vi "daq.io Machine Example.vi"(8 "error in":errorcluster) -> (0 "error out":errorcluster)   [LabVIEW 2013, in "daqio minimal.lvlib"]
doc: "This interactive example demonstrates how a device or machine could continuously publish data to daq.io. When correct user credentials are given, it will log on to daq.io, autocreate all device settings if required and will update time series values continuously. When changing the tag values (or Tags), these will be updated as well. When firing an Event, it will become visible on the daq.io events page. \n\nRefer to the Embedded example for an example that can easily be run on a RIO platform continuously."
uses:
  daqio minimal.lvlib
  _typedefs/update-button.ctl
  _typedefs/trigger-button.ctl
  _typedefs/exmpl_overlay_mask.ctl
  _typedefs/dashboard-button.ctl
  _typedefs/waveform-button.ctl
  _typedefs/exmpl-states.ctl
  _typedefs/daqio-Credentials.ctl
  _typedefs/daqio-Type.ctl
  <vilib>/httpClient/ClientHandle.ctl
  <vilib>/Platform/browser.llb/Open URL in Default Browser (string).vi
  _subs/daqio_Write_Multiple_single_Timestamp.vi
  _subs/daqio_Write_Waveform.vi
  <vilib>/httpClient/LabVIEWHTTPClient.lvlib
  <vilib>/measure/NI_MABase.lvlib
panel:
  out "overlay mask":T1
  in  "Create Waveform":T2
  in  "Create Dashboard":T3
  out "Log":string[](array[string])
  in  "Stop":bool
  in  "Fire Event":T4
  in  "Select Event":u16(ring) items=["Safety Hood Status", "Manual Operation", "Shutting Down"]
  out "Time Stamp sent":timestamp
  in  "Event Data":string
  in  "Update Tags":T5
  out "connected to daq.io":bool
  in  "Sign up link":bool caption="Boolean"
  out "Speed (RPM)":dbl(knob) scale=0.0..2000.0
  out "Temperature Data":dbl(graph)
  out "RAM":dbl(slide) scale=0.0..100.0
  out "CPU":dbl(slide) scale=0.0..100.0
  in  "Setpoint\n(set manually)":dbl(knob) scale=0.0..100.0
  in  "Value 3":string="1234-abc"
  in  "Value 2":string="XYZ 3000 Plus"
  in  "Tag 3":string="Serial Number"
  in  "Tag 2":string="Type"
  in  "Value 1":string="47.615459, -122.323804"
  in  "Tag 1":string="Location"
  out "Device Key":string
  in  "Log On":bool
  in  "User Name (your email)":string
  in  "Password":string
  out "Dashboard URL - copy and open in your web browser":string
  # "Get your free account at daq.io first: sign up at"
  # "This Machine"
  # "(autogenerated in this example)"
  # "Device Tags"
  # "Use device tags to describe \nspecific parameters for each\ndevice. These can include the \nlocation, the serial number or\nother machine or location-\nspecific information. These\nfields are fully user-defined."
  # "Device Events"
  # "Use device events to signal\nany local event to daq.io. These\ncould include mechanical events\n(e.g. \"safety latch released\") or \nany change on the device that\nneeds to be tracked."
  # "Device Live Data Channels"
  # "Use device channels to transfer\ntime series data. All channels \nof the device will be visible in \nthe online data viewer. You \ncan build your own dashboard \nin the webbrowser and link it\nto exisiting channels. Clicking\n\"Create Dashboard\" will\ngenerate a dashboard \nfor this example."
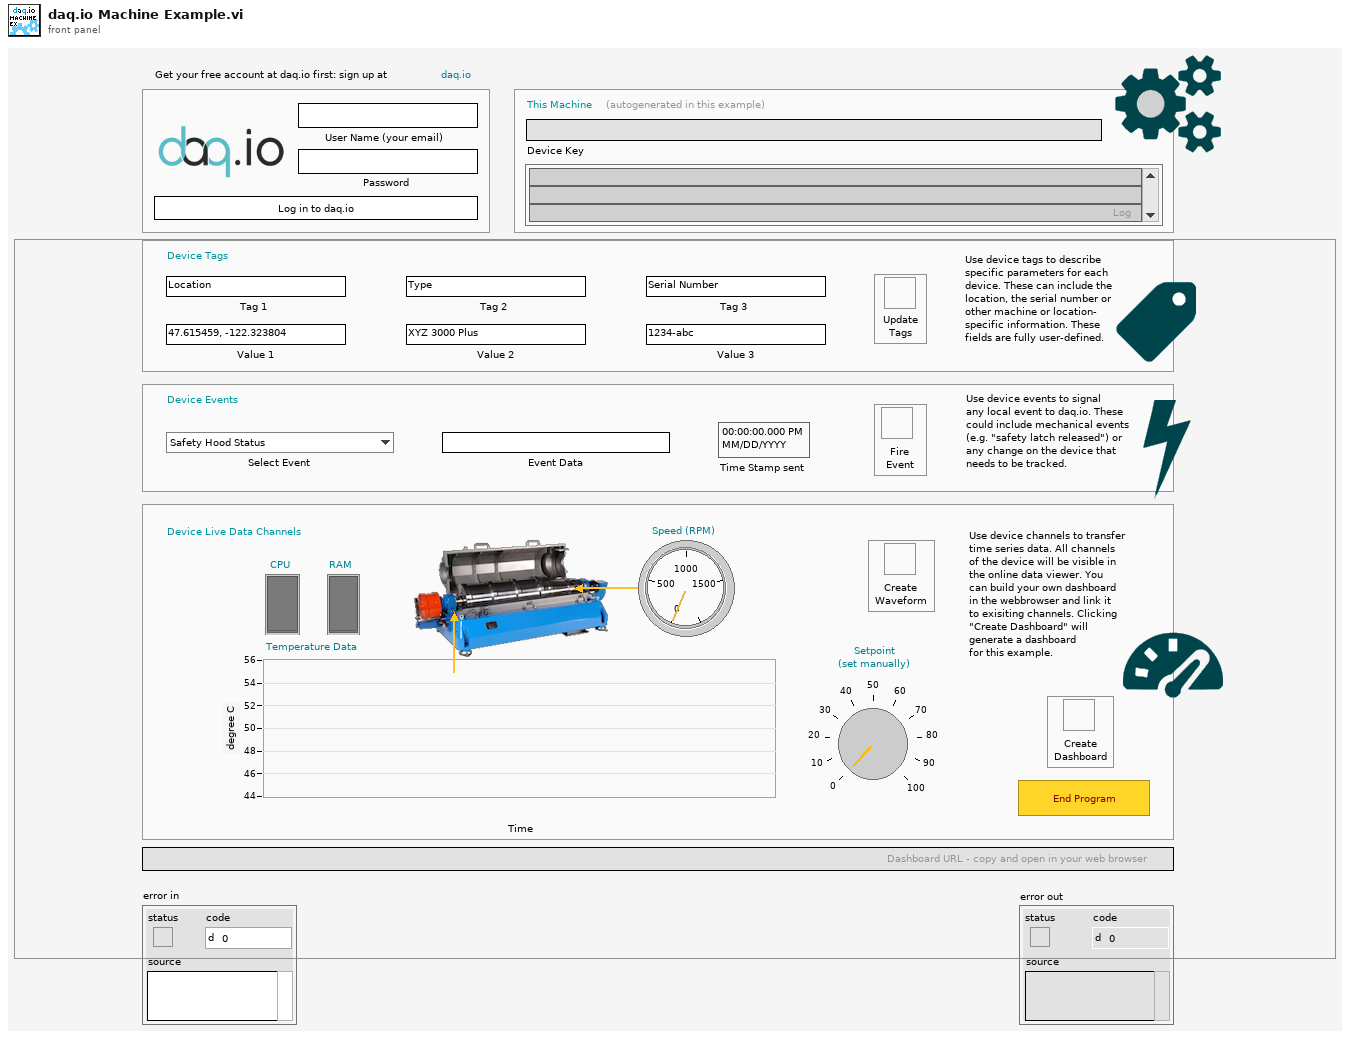
[diagram p1: front panel]
types:
  T1 = typedef "daqio minimal.lvlib/exmpl_overlay_mask.ctl" = bool
  T2 = typedef "daqio minimal.lvlib/waveform-button.ctl" = bool
  T3 = typedef "daqio minimal.lvlib/dashboard-button.ctl" = bool
  T4 = typedef "daqio minimal.lvlib/trigger-button.ctl" = bool
  T5 = typedef "daqio minimal.lvlib/update-button.ctl" = bool
  T6 = typedef "daqio minimal.lvlib/exmpl-states.ctl" = enum16{"idle", "time series", "fire events", "update tags", "end program", "create waveform", "create dashboard"}
  T7 = typedef "daqio minimal.lvlib/daqio-Credentials.ctl" = cluster{"User Name (email)":string, "Password":string}
  T8 = typedef "daqio minimal.lvlib/daqio-Type.ctl" = cluster{"daq.io ref":T9, "daq.io API Base":string, "Device Key":string, "Account ID":string, "online":bool, "SSL":bool, "buffer":bool}
  T9 = typedef "LabVIEWHTTPClient.lvlib/ClientHandle.ctl" = refnum<k1>
  T10 = enum8{"Enabled", "Disabled", "Disabled and Grayed Out"}
  T11 = enum16{"Sine Wave", "Triangle Wave", "Square Wave", "Sawtooth Wave"}
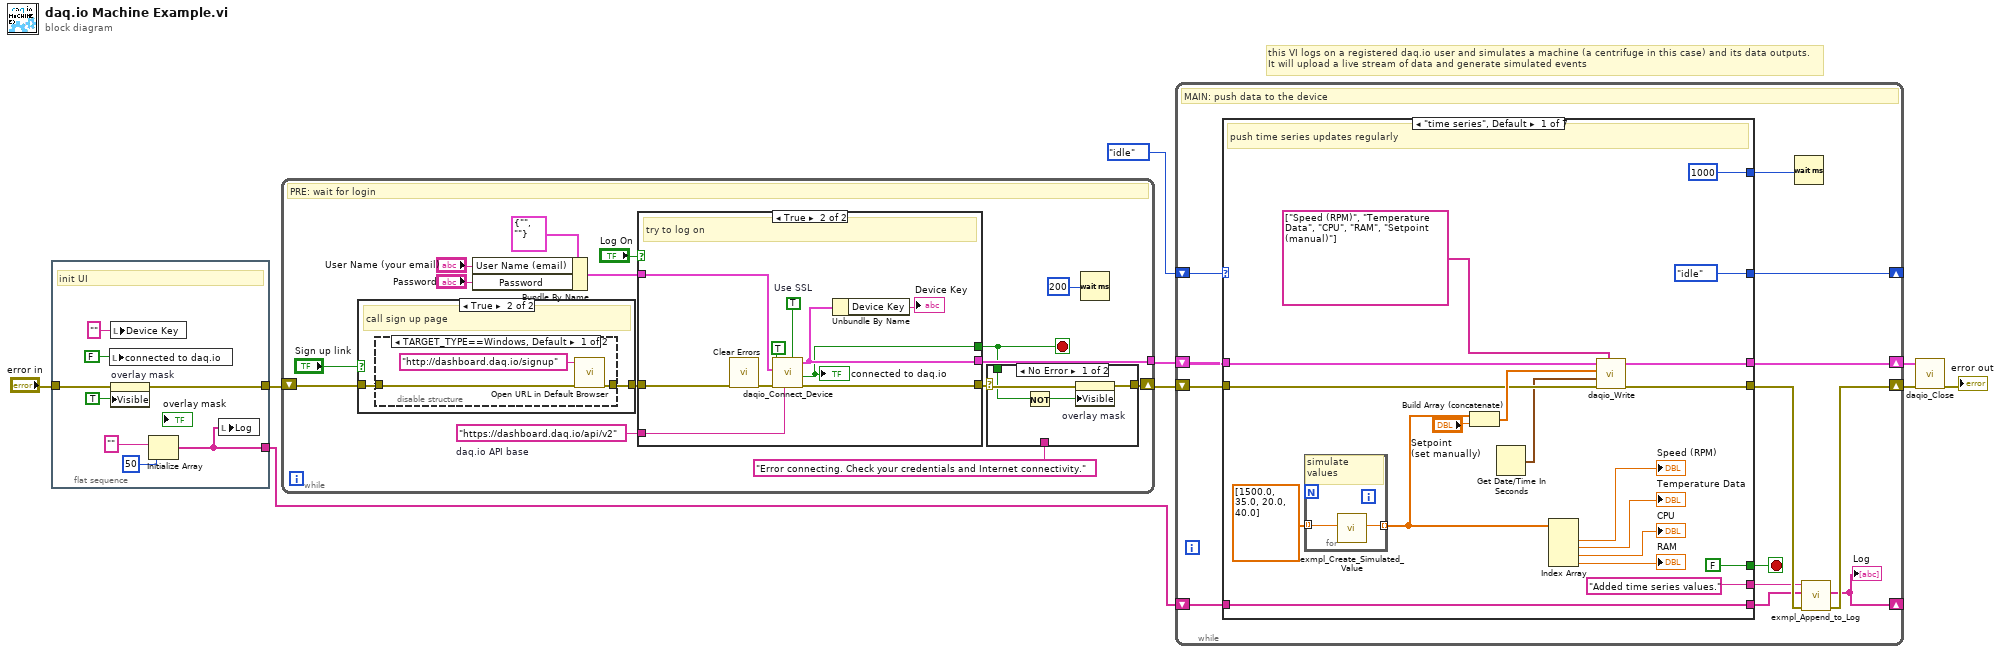
[diagram p0: block diagram]
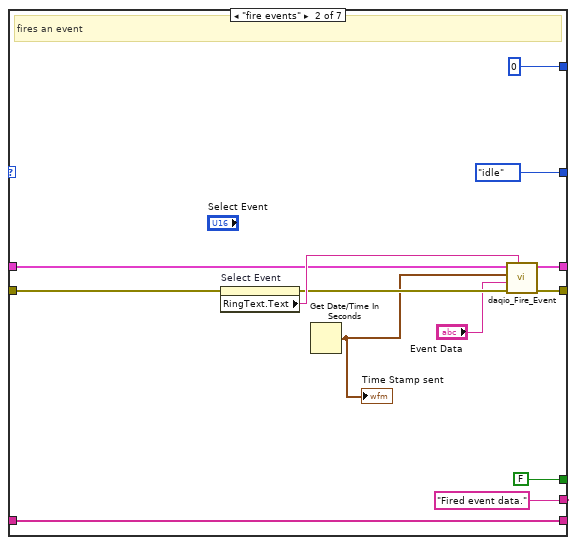
[diagram p2: hidden frame]
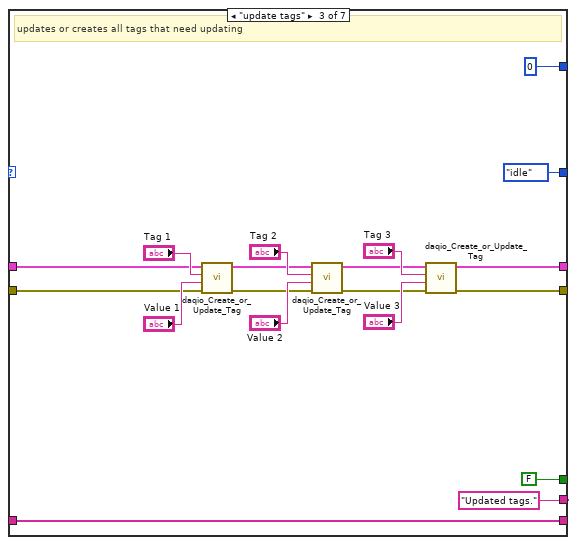
[diagram p3: hidden frame]
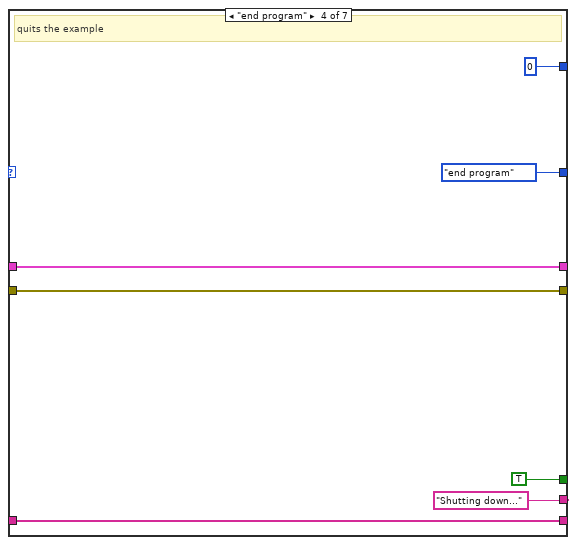
[diagram p4: hidden frame]
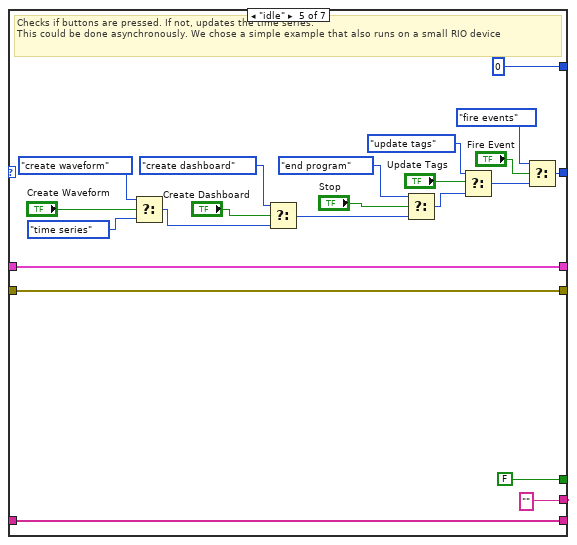
[diagram p5: hidden frame]
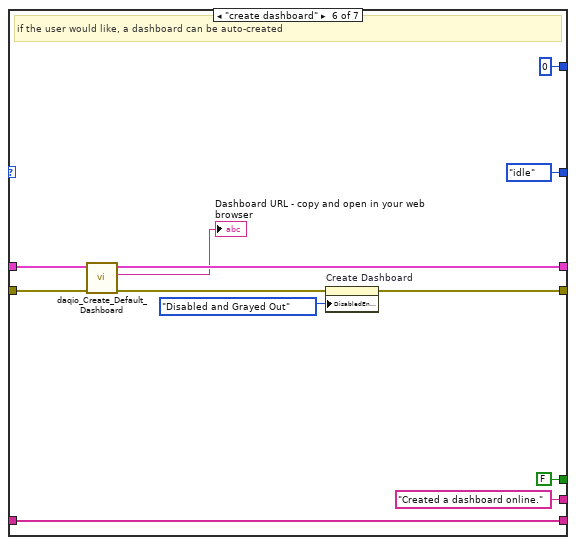
[diagram p6: hidden frame]
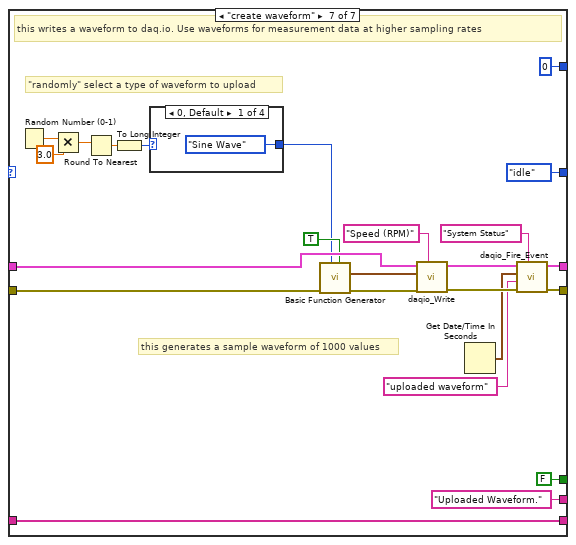
[diagram p7: hidden frame]
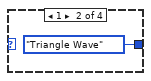
[diagram p8: hidden frame]
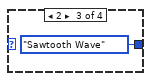
[diagram p9: hidden frame]
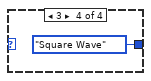
[diagram p10: hidden frame]
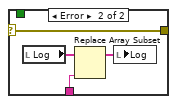
[diagram p11: hidden frame]
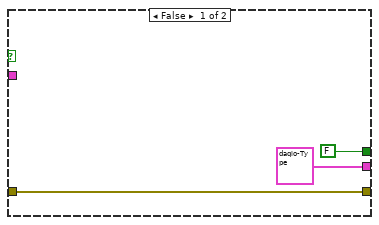
[diagram p14: hidden frame]
diagram:
  # "this VI logs on a registered daq.io user and simulates a machine (a centrifuge in this case) and its data outputs. \nIt will upload a live stream of data and generate simulated events"
  n1 = flat-sequence {
    tunnel: [w14] -> w6
    tunnel: "error in" -> [w15]
    tunnel: [w10] -> w1
    frame #0 {
      # "init UI"
      n2 = local write "connected to daq.io"(FALSE ("connected to daq.io")) -> ()
      n3 = local write "Device Key"("" ("log")) -> ()
      n4 = property on="overlay mask" class="Bool (strict)"(error in=w15, "Visible"=TRUE) -> (error out=w14:errorcluster)  [unwired: 1 in, 1 out]
      n5 = Initialize Array("" ("log"), 50 ("dimension size")) -> (w10:string[])
      n6 = local write "Log"(w10) -> ()
    }
  }
  n7 = while {
    shift-right: [w20] -> w4
    shift-left: w6 -> [w25]
    tunnel: [w27] -> w5
    stop <- w19 stop-if-true
    w18 = "https://dashboard.daq.io/api/v2"  # daq.io API base
    # "PRE: wait for login"
    n8 = case shown="True" "Sign up link" {
      tunnel: w25 -> [w41 w43]
      tunnel: [w41 w42] -> w24
      frame False {
      }
      frame True {
        # "call sign up page"
        n9 = disable-structure shown="TARGET_TYPE==Windows, Default" {
          disable-tunnel: w43 -> [w45 w47]
          disable-tunnel: [w44 w47] -> w42
          frame condition #0 (active) {
            n10 = call-poly <vilib>:"Open URL in Default Browser.vi"("error in (no error)"=w45, "URL"="http://dashboard.daq.io/signup") -> ("error out"=w44:errorcluster)  [unwired: 4 in, 1 out]
          }
          frame condition #1 {
          }
        }
      }
    }
    n11 = Bundle By Name(cluster=T7 {"User Name (email)"="", "Password"=""} ("daq.io Credentials"), "User Name (email)"="User Name (your email)", "Password"="Password") -> (w26:T7)
    n12 = case shown="True" "Log On" {
      tunnel: [T8 {"daq.io ref"=refnum, "daq.io API Base"="http://dashboard.daq.io/api/v1", "Device Key"="", "Account ID"="", "online"=FALSE, "SSL"=FALSE, "buffer"=FALSE} ("daq.io type out") w57] -> w27
      tunnel: [w48 w60] -> w21
      tunnel: w24 -> [w48 w59]
      tunnel: w18 -> [_ w58]
      tunnel: w26 -> [_ w51]
      tunnel: [FALSE ("connected successfully?") w55] -> w19
      frame False {
      }
      frame True {
        w52 = TRUE  # Use SSL
        # "try to log on"
        n13 = call <vilib>:"Clear Errors.vi"("error in (no error)"=w59) -> ("error out"=w54:errorcluster)  [unwired: 6 in]
        n14 = call "daqio_Connect_Device.vi"("Use SSL"=w52, "daq.io API base"=w58, "error in (no error)"=w54, "Credentials"=w51, "Use System Status Event?"=TRUE) -> ("error out"=w60:errorcluster, "connected successfully?"=w55:bool, "daq.io type out"=w57:T8)  [unwired: 4 in]
        "connected to daq.io" <- w55
        n15 = Unbundle By Name(w57) -> ("Device Key"=→"Device Key":string)
      }
    }
    n16 = case shown="No Error" w21 {
      selector: w21 -> [w35 w37]
      tunnel: "Error connecting. Check your credentials and Internet connectivity." ("new element/subarray") -> [_ w38]
      tunnel: [w36 w37] -> w20
      tunnel: w19 -> [w34 _]
      frame No Error {
        n17 = Not(x=w34) -> (.not. x?=w33:bool)
        n18 = property on="overlay mask" class="Bool (strict)"(error in=w35, "Visible"=w33) -> (error out=w36:errorcluster)  [unwired: 1 in, 1 out]
      }
      frame Error {
        n19 = local read "Log"() -> (w40:string[])
        n20 = Replace Array Subset(array=w40, new element=w38) -> (w39:string[])  [unwired: 1 in]
        n21 = local write "Log"(w39) -> ()
      }
    }
    n22 = Wait (ms)(milliseconds to wait=u32 200) -> ()  [unwired: 1 out]
  }
  n23 = while {
    shift-right: [w64] -> w9
    shift-left: w4 -> [w72]
    shift-right: [w71] -> w3
    shift-left: w5 -> [w73]
    shift-right: [w69] -> _
    shift-left: exmpl-states."idle" -> [w70]
    shift-right: [w61] -> _
    shift-left: w1 -> [w66]
    stop <- w68 stop-if-true
    # "MAIN: push data to the device"
    n24 = case shown="\"time series\", Default" w70 {
      tunnel: w73 -> [w80 w104 w116 w131 w136 w162 w190]
      tunnel: w72 -> [w77 w103 w115 w130 w135 w161 w187]
      tunnel: [w74 w101 w113 w131 w136 w160 w180] -> w71
      tunnel: [w75 w102 w114 w130 w135 w157 w179] -> w65
      tunnel: [exmpl-states."idle" exmpl-states."idle" exmpl-states."idle" exmpl-states."end program" w152 exmpl-states."idle" exmpl-states."idle"] -> w69
      tunnel: [FALSE FALSE FALSE TRUE FALSE FALSE FALSE] -> w68
      tunnel: [u32 1000 ("milliseconds to wait") u32 0 ("milliseconds to wait") u32 0 ("milliseconds to wait") u32 0 ("milliseconds to wait") u32 0 ("milliseconds to wait") u32 0 ("milliseconds to wait") u32 0 ("milliseconds to wait")] -> w67
      tunnel: ["Added time series values." ("log") "Fired event data." ("log") "Updated tags." ("log") "Shutting down..." ("log") "" ("log") "Created a dashboard online." ("log") "Uploaded Waveform." ("log")] -> w63
      tunnel: w66 -> [w82 w96 w108 w127 w144 w167 w191]
      tunnel: [w82 w96 w108 w127 w144 w167 w191] -> w62
      frame "time series", Default {
        # "push time series updates regularly"
        n25 = for {
          tunnel: [w94] -> w91 mode=indexing
          tunnel: dbl[] [1500.0, 35.0, 20.0, 40.0] -> [w93] mode=indexing
          # "simulate\nvalues"
          n26 = call "exmpl_Create_Simulated_Value.vi"("offset"=w93) -> ("Numeric"=w94:dbl)  [unwired: 9 in, 1 out]
        }
        n27 = Build Array (concatenate)(w91, "Setpoint\n(set manually)") -> (w78:dbl[])
        n28 = Get Date/Time In Seconds() -> (seconds since 1Jan1904=w76:timestamp)
        n29 = Index Array(array=w91) -> (element #1=→"Speed (RPM)":dbl, element #2=→"Temperature Data":dbl, element #3=→"CPU":dbl, element #4=→"RAM":dbl)  [unwired: 4 in]
        n30 = call-poly "daqio_Write.vi"("daq.io Device Channel Keys"=string[] ["Speed (RPM)", "Temperature Data", "CPU", "RAM", "Setpoint (manual)"], "error in (no error)"=w77, "Timestamp"=w76, "Values"=w78, "daq.io type in"=w80) -> ("error out"=w75:errorcluster, "daq.io type out"=w74:T8)  [unwired: 5 in]
      }
      frame "fire events" {
        # "fires an event"
        n31 = property on="Select Event" class="Ring (strict)"(error in=w103) -> (error out=w106:errorcluster, "RingText.Text"=w107:string)  [unwired: 1 in, 1 out]
        n32 = Get Date/Time In Seconds() -> (seconds since 1Jan1904=w95:timestamp)
        "Time Stamp sent" <- w95
        n33 = call "daqio_Fire_Event.vi"("Event Key"=w107, "error in (no error)"=w106, "Event Value"="Event Data", "Event Date and Time"=w95, "daq.io type in"=w104) -> ("error out"=w102:errorcluster, "daq.io type out"=w101:T8)  [unwired: 5 in]
      }
      frame "update tags" {
        # "updates or creates all tags that need updating"
        n34 = call "daqio_Create_or_Update_Tag.vi"("error in (no error)"=w115, "Tag Value"="Value 1", "Tag Key"="Tag 1", "daq.io type in"=w116) -> ("error out"=w120:errorcluster, "daq.io type out"=w117:T8)  [unwired: 5 in, 1 out]
        n35 = call "daqio_Create_or_Update_Tag.vi"("error in (no error)"=w120, "Tag Value"="Value 2", "Tag Key"="Tag 2", "daq.io type in"=w117) -> ("error out"=w119:errorcluster, "daq.io type out"=w118:T8)  [unwired: 5 in, 1 out]
        n36 = call "daqio_Create_or_Update_Tag.vi"("error in (no error)"=w119, "Tag Value"="Value 3", "Tag Key"="Tag 3", "daq.io type in"=w118) -> ("error out"=w114:errorcluster, "daq.io type out"=w113:T8)  [unwired: 5 in, 1 out]
      }
      frame "end program" {
        # "quits the example"
      }
      frame "idle" {
        # "Checks if buttons are pressed. If not, updates the time series. \nThis could be done asynchronously. We chose a simple example that also runs on a small RIO device"
        n37 = Select(t=exmpl-states."create waveform", s="Create Waveform", f=exmpl-states."time series") -> (s? t:f=w138:T6)
        n38 = Select(t=exmpl-states."create dashboard", s="Create Dashboard", f=w138) -> (s? t:f=w141:T6)
        n39 = Select(t=exmpl-states."end program", s="Stop", f=w141) -> (s? t:f=w146:T6)
        n40 = Select(t=exmpl-states."update tags", s="Update Tags", f=w146) -> (s? t:f=w153:T6)
        n41 = Select(t=exmpl-states."fire events", s="Fire Event", f=w153) -> (s? t:f=w152:T6)
      }
      frame "create dashboard" {
        # "if the user would like, a dashboard can be auto-created"
        n42 = call "daqio_Create_Default_Dashboard.vi"("error in"=w161, "daq.io type in"=w162) -> ("error out"=w158:errorcluster, "Dashboard URL"=→"Dashboard URL - copy and open in your web browser":string, "daq.io type out"=w160:T8)  [unwired: 7 in]
        n43 = property on="Create Dashboard" class="Bool"(error in=w158, "DisabledEnum"=T10."Disabled and Grayed Out" ("Disabled")) -> (error out=w157:errorcluster)  [unwired: 1 in, 1 out]
      }
      frame "create waveform" {
        # "\"randomly\" select a type of waveform to upload"
        # "this generates a sample waveform of 1000 values"
        # "this writes a waveform to daq.io. Use waveforms for measurement data at higher sampling rates"
        n44 = Random Number (0-1)() -> (number: 0 to 1=w173:dbl)
        n45 = Multiply(x=w173, y=3.0) -> (x*y=w171:dbl)
        n46 = Round To Nearest(number=w171) -> (nearest integer value=w170:dbl)
        n47 = To Long Integer(number=w170) -> (32bit integer=w169:i32)
        n48 = case shown="0, Default" w169 {
          tunnel: [T11."Sine Wave" ("signal type") T11."Triangle Wave" ("signal type") T11."Sawtooth Wave" ("signal type") T11."Square Wave" ("signal type")] -> w168
          frame 0, Default {
          }
          frame 1 {
          }
          frame 2 {
          }
          frame 3 {
          }
        }
        n49 = call <vilib>:"Basic Function Generator.vi"("reset signal"=TRUE, "signal type"=w168, "error in (no error)"=w187) -> ("error out"=w189:errorcluster, "signal out"=w188:waveform(dbl))  [unwired: 6 in, 1 out]
        n50 = call-poly "daqio_Write.vi"("daq.io Device Channel Key"="Speed (RPM)" ("daq.io Device Channel"), "error in (no error)"=w189, "Waveform"=w188, "daq.io type in"=w190) -> ("error out"=w178:errorcluster, "daq.io type out"=w181:T8)  [unwired: 6 in]
        n51 = Get Date/Time In Seconds() -> (seconds since 1Jan1904=w177:timestamp)
        n52 = call "daqio_Fire_Event.vi"("Event Key"="System Status", "error in (no error)"=w178, "Event Value"="uploaded waveform", "Event Date and Time"=w177, "daq.io type in"=w181) -> ("error out"=w179:errorcluster, "daq.io type out"=w180:T8)  [unwired: 5 in]
      }
    }
    n53 = Wait (ms)(milliseconds to wait=w67) -> ()  [unwired: 1 out]
    n54 = call "exmpl_Append_to_Log.vi"("error in (no error)"=w65, "Log Array in"=w62, "Log Message"=w63) -> ("error out"=w64:errorcluster, "Log Array out"=w61:string[])  [unwired: 7 in]
    "Log" <- w61
  }
  n55 = call "daqio_Close.vi"("error in (no error)"=w9, "daq.io type"=w3) -> ("error out"=→"error out":errorcluster)  [unwired: 9 in]
